vi "CvrtCell2Data.vi"(8 "error in (no error)":errorcluster, 9 "Header Names":T1, 10 "Item Name":string, 11 "Channel in":refnum<class "Channel.lvclass">) -> (0 "error out":errorcluster, 3 "Channel out":refnum<class "Channel.lvclass">)   [LabVIEW 2018, in "Measurement Channels.lvlib" / "Channel.lvclass"]
uses:
  Channel.lvclass
  Common/Controls/HeaderNames.ctl
  Channel.lvclass/Channel.ctl
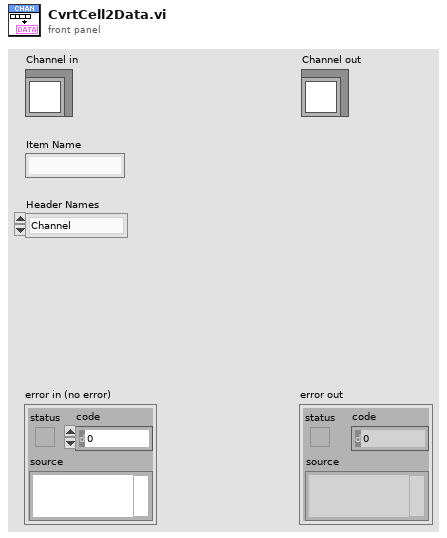
[diagram p1: front panel]
types:
  T1 = typedef "HeaderNames.ctl" = enum16{"Channel", "Device", "Spacer", "Description", "MB", "Range", "Terminal", "Coupling", "Thresh (V)", "Pulse/Rev", "Slope", "Min EU", "Min RPM", "mV/EU", "Iex", "Temp Units", "Type", "CJC Src", "CJC Val", "Ro", "Wire Cfg", "Strain Mode", "Vex", "Bridge Type", "GF", "Gauge Res", "Poisson", "Lead Res", "Init Strain", "GAF", "Scale", "Offset", "Unit (EU)", "dB?", "dB Ref", "Cal Mag", "Cal Units", "Max Temp", "Min Temp", "Max Strain", "Min Strain"}
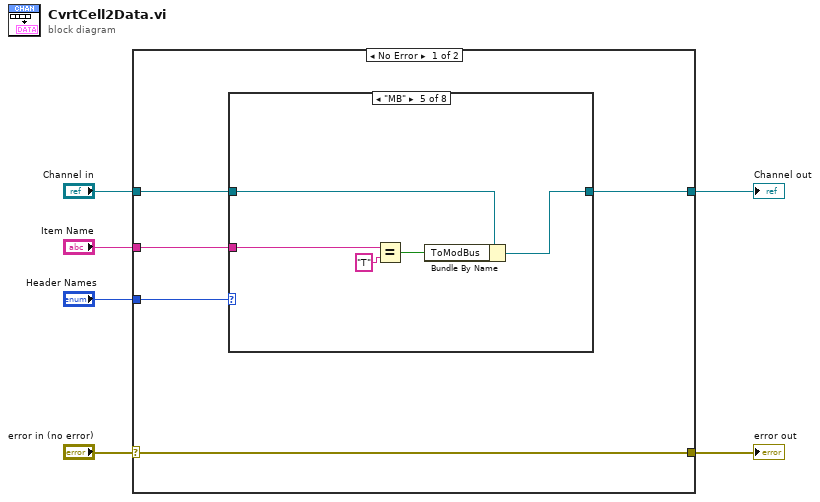
[diagram p0: block diagram]
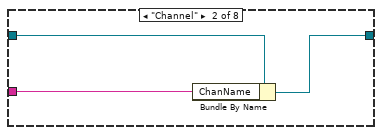
[diagram p3: hidden frame]
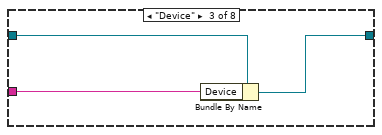
[diagram p4: hidden frame]
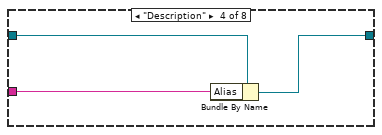
[diagram p5: hidden frame]
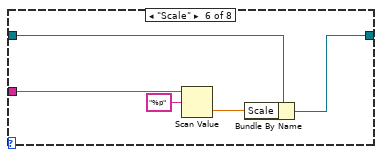
[diagram p6: hidden frame]
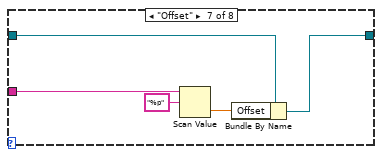
[diagram p7: hidden frame]
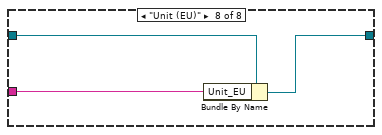
[diagram p8: hidden frame]
diagram:
  n1 = case shown="No Error" "error in (no error)" {
    selector: "error in (no error)" -> [w11 w41]
    tunnel: [w11 w41] -> w5
    tunnel: [w10 w40] -> w3
    tunnel: "Channel in" -> [w8 w40]
    tunnel: "Item Name" -> [w9 _]
    tunnel: "Header Names" -> [w7 _]
    frame No Error {
      n2 = case shown="\"MB\"" w7 {
        tunnel: w9 -> [_ w13 w16 w19 w25 w29 w33 w38]
        tunnel: w8 -> [w12 w15 w18 w21 w24 w31 w36 w39]
        tunnel: [w12 w14 w17 w20 w23 w30 w35 w37] -> w10
        frame Default {
        }
        frame "Channel" {
          n3 = Bundle By Name(cluster=w15, "ChanName"=w13) -> (w14:refnum<class "Channel.lvclass">)
        }
        frame "Device" {
          n4 = Bundle By Name(cluster=w18, "Device"=w16) -> (w17:refnum<class "Channel.lvclass">)
        }
        frame "Description" {
          n5 = Bundle By Name(cluster=w21, "Alias"=w19) -> (w20:refnum<class "Channel.lvclass">)
        }
        frame "MB" {
          n6 = Equal?(x=w25, y="T") -> (x = y?=w22:bool)
          n7 = Bundle By Name(cluster=w24, "ToModBus"=w22) -> (w23:refnum<class "Channel.lvclass">)
        }
        frame "Scale" {
          n8 = Scan Value(string=w29, format string="%p") -> (value=w27:dbl)  [unwired: 1 in, 1 out]
          n9 = Bundle By Name(cluster=w31, "Scale"=w27) -> (w30:refnum<class "Channel.lvclass">)
        }
        frame "Offset" {
          n10 = Scan Value(string=w33, format string="%p") -> (value=w32:dbl)  [unwired: 1 in, 1 out]
          n11 = Bundle By Name(cluster=w36, "Offset"=w32) -> (w35:refnum<class "Channel.lvclass">)
        }
        frame "Unit (EU)" {
          n12 = Bundle By Name(cluster=w39, "Unit_EU"=w38) -> (w37:refnum<class "Channel.lvclass">)
        }
      }
    }
    frame Error {
    }
  }
  "error out" <- w5
  "Channel out" <- w3
